vi "MD5 Encrypt.vi"(8 "error in (no error)":errorcluster, 11 "data":string) -> (0 "error out":errorcluster, 3 "encrypted data":string)   [LabVIEW 2023, in "MD5.lvclass"]
uses:
  MD5.lvclass
panel:
  out "MD5 out":refnum<class "MD5.lvclass">
  in  "MD5 in":refnum<class "MD5.lvclass">
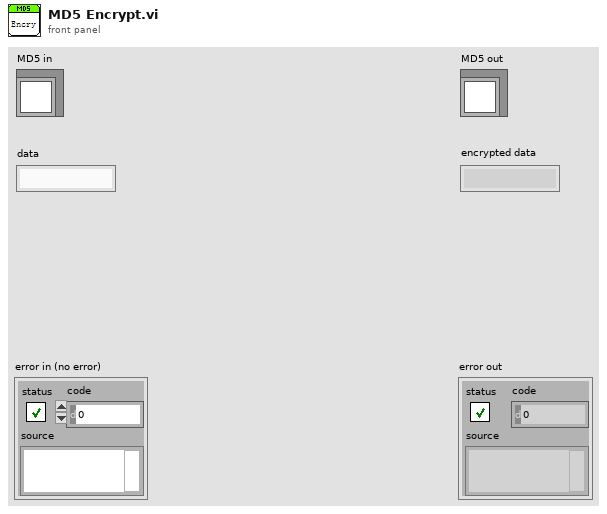
[diagram p1: front panel]
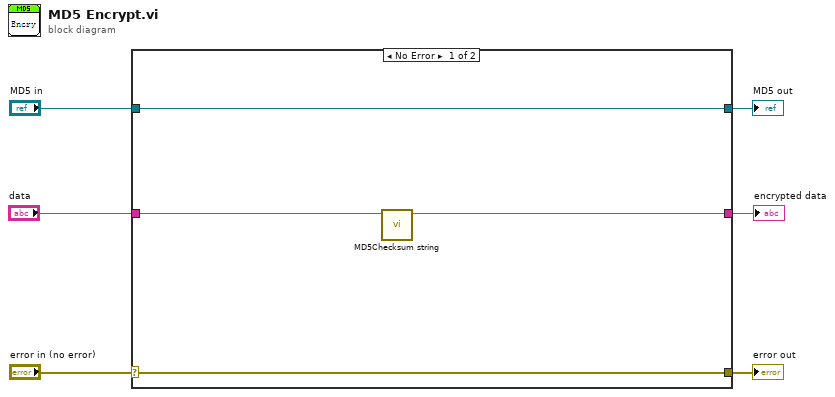
[diagram p0: block diagram]
diagram:
  n1 = case shown="No Error" "error in (no error)" {
    selector: "error in (no error)" -> [w9 w12]
    tunnel: [w9 w12] -> w5
    tunnel: [w10 w11] -> w3
    tunnel: "MD5 in" -> [w10 w11]
    tunnel: "data" -> [w8 _]
    tunnel: [w7 _] -> w1
    frame No Error {
      n2 = call <vilib>:"MD5Checksum string.vi"("Message String"=w8) -> ("MD5 message-digest"=w7:string)  [unwired: 10 in]
    }
    frame Error {
    }
  }
  "error out" <- w5
  "MD5 out" <- w3
  "encrypted data" <- w1
